vi "12.2-LabelSegment.vi"() -> ()   [LabVIEW 2016]
doc: "This example shows how to label a binary image that contains multiple particles. The labeling process assigns a unique value to all the pixels that belong to a particle. Some processing functions in NI Vision require the input binary image to be labeled."
uses:
  <vilib>/vision/NI_Vision_Development_Module.lvlib
panel:
  out "Index of Extracted Particles":i32
  out "Particle Extracted":T1(plugin-control)
  out "Seg":T1(plugin-control)
  out "Labeled":T1(plugin-control)
  out "Region Reports":T2(array[cluster]) {"Mean Value" format="%.2f"; "%" format="%.2f"; "Area (calibrated)" format="%.2f"; "Maximal Value" format="%.2f"; "Minimal Value" format="%.2f"; "Standard Variation" format="%.2f"}
  out "Original":T1(plugin-control)
  out "# of Particles":i32
  in  "Threshold Values":T3(slide)={"Minimum Value"=117.55319, "Maximum Value"=255.0} scale=0.0..255.0
  in  "Connectivity":bool
  # "Tips:\n1) Change the Threshold values to see the Labeled image. \n2) Each distinct particle is labeled with a different pixel value which gives each particle a different color.\n3) Use Binary Palette for Labeled image control"
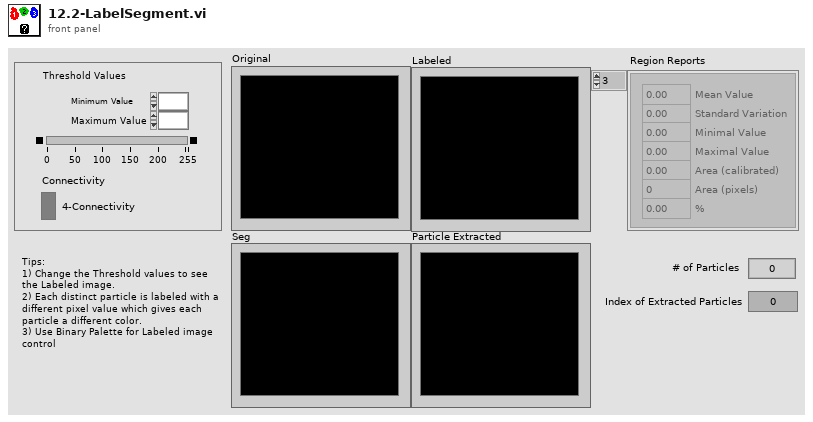
[diagram p1: front panel]
types:
  T1 = typedef "IMAQ Image.ctl" = refnum<image>
  T2 = cluster{"Mean Value":sgl, "Standard Variation":sgl, "Minimal Value":sgl, "Maximal Value":sgl, "Area (calibrated)":sgl, "Area (pixels)":i32, "%":sgl}[]
  T3 = cluster{"Minimum Value":sgl, "Maximum Value":sgl}
  T4 = enum32{"AutoM", "Close", "Dilate", "Erode", "Gradient", "Gradient out", "Gradient in", "Hit miss", "Open", "PClose", "POpen", "Thick", "Thin"}
  T5 = cluster{"Mean Value":sgl, "Standard Variation":sgl, "Minimal Value":sgl, "Maximal Value":sgl, "Area (calibrated)":sgl, "Area (pixels)":i32, "%":sgl}
  T6 = typedef "ROI Descriptor" = cluster{"Global Rectangle":i32[], "Contours":cluster{"ID":enum32{"External", "Internal"}, "Type":u32, "Coordinates":i32[]}[]}
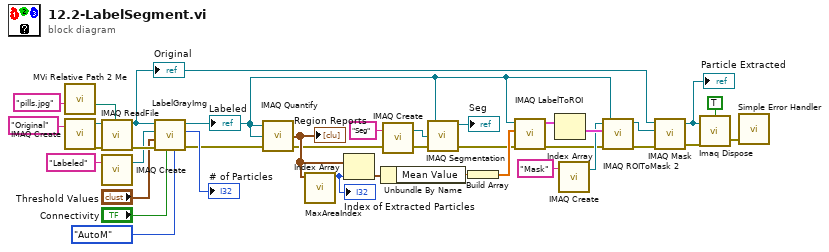
[diagram p0: block diagram]
diagram:
  n1 = call "MVi Relative Path 2 Me.vi"("Relative Path"="pills.jpg" ("name or relative path")) -> ("Appended Dir"=w32:path)  [unwired: 5 in, 1 out]
  n2 = call "IMAQ Create"("Image Name"="Original") -> ("New Image"=w34:T1, "error out"=w35:errorcluster)  [unwired: 4 in]
  n3 = call "IMAQ ReadFile"("File Path"=w32, "error in (no error)"=w35, "Image"=w34) -> ("error out"=w26:errorcluster, "Image Out"=w4:T1)  [unwired: 4 in, 3 out]
  "Original" <- w4
  n4 = call "IMAQ Create"("Image Name"="Labeled") -> ("New Image"=w25:T1)  [unwired: 4 in, 1 out]
  n5 = call "LabelGrayImg.vi"("Operation"=T4."AutoM", "Connectivity"="Connectivity", "EorIn"=w26, "Threshold Values"="Threshold Values", "Dst"=w25, "Src"=w4) -> ("ErrOut"=w18:errorcluster, "# of Particles found"=→"# of Particles":i32, "ImgOut"=w2:T1)  [unwired: 3 in]
  "Labeled" <- w2
  n6 = call "IMAQ Quantify"("error in (no error)"=w18, "Image Mask"=w2, "Image"=w2) -> ("error out"=w8:errorcluster, "Region Reports"=w12:T2)  [unwired: 1 out]
  "Region Reports" <- w12
  n7 = call "MaxAreaIndex.vi"("Region Reports"=w12) -> ("Index"=w11:i32)  [unwired: 10 in]
  "Index of Extracted Particles" <- w11
  n8 = Index Array(array=w12, index=w11) -> (element=w15:T5)
  n9 = Unbundle By Name(w15) -> ("Mean Value"=w14:sgl)
  n10 = call "IMAQ Create"("Image Name"="Seg", "error in (no error)"=w8) -> ("New Image"=w3:T1, "error out"=w9:errorcluster)  [unwired: 3 in]
  n11 = call "IMAQ Segmentation"("error in (no error)"=w9, "Image Dst"=w3, "Image Src"=w2) -> ("error out"=w7:errorcluster, "Image Dst Out"=→"Seg":T1)  [unwired: 1 in]
  n12 = Build Array(w14) -> (w13:sgl[])
  n13 = call "IMAQ LabelToROI"("error in (no error)"=w7, "Labels In"=w13, "Image"=w2) -> ("error out"=w1:errorcluster, "ROIs"=w29:T6[])  [unwired: 5 in, 2 out]
  n14 = Index Array(array=w29) -> (element=w28:T6)  [unwired: 1 in]
  n15 = call "IMAQ Create"("Image Name"="Mask") -> ("New Image"=w27:T1)  [unwired: 4 in, 1 out]
  n16 = call "IMAQ ROIToMask 2"("Image Model"=w2, "error in (no error)"=w1, "ROI Descriptor"=w28, "Image"=w27) -> ("error out"=w16:errorcluster, "Image Out"=w17:T1)  [unwired: 5 in, 1 out]
  n17 = call "IMAQ Mask"("error in (no error)"=w16, "Image Mask"=w17, "Image Src"=w4) -> ("error out"=w5:errorcluster, "Image Dst Out"=w10:T1)  [unwired: 2 in]
  "Particle Extracted" <- w10
  n18 = call "Imaq Dispose"("All Images? (No)"=TRUE, "Image"=w10, "error in (no error)"=w5) -> ("error out"=w19:errorcluster)  [unwired: 3 in]
  n19 = call <vilib>:"Simple Error Handler.vi"("error in (no error)"=w19) -> ()  [unwired: 4 in, 5 out]
